vi "OAT Demodulate Order.vi"   [LabVIEW 2017, in "SoundVib_Resampling.lvlib"]
uses:
  <vilib>/addons/Sound and Vibration/Order Analysis/Resample Order Tracking/SoundVib_Resampling.lvlib
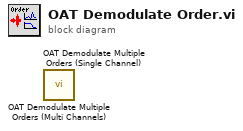
[diagram p0: block diagram]
diagram:
  n1 = call <vilib>:"OAT Demodulate Multiple Orders (Multi Channels).vi"() -> ()  [unwired: 11 in, 5 out]
  n2 = call <vilib>:"OAT Demodulate Multiple Orders (Single Channel).vi"() -> ()  [unwired: 11 in, 5 out]
